vi "Set Gamma Adjust.vi"(8 "error in (no error)":errorcluster, 9 "Gamma Adjust":dbl=120.0, 10 "CAN Offset":u32=160 format="%x", 11 "interface object in":refnum<k20>) -> (0 "error out":errorcluster, 3 "interface object out":refnum<k20>)   [LabVIEW 2014]
uses:
  <vilib>/RioEmbeddedCAN/RioEmbeddedCAN.llb/CANWrite.vi
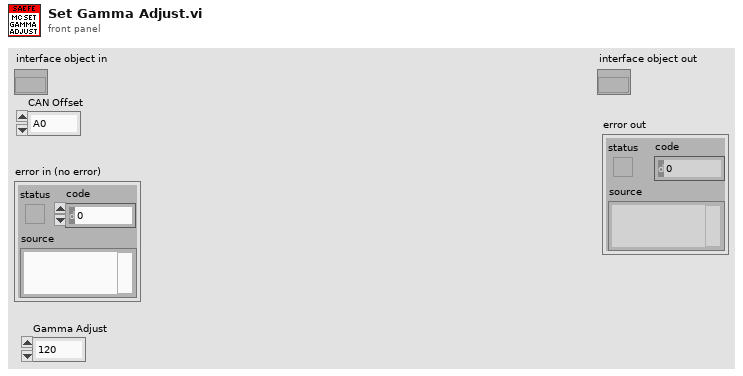
[diagram p1: front panel]
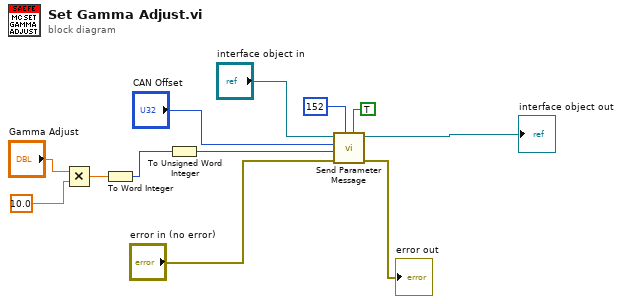
[diagram p0: block diagram]
diagram:
  n1 = Multiply(x="Gamma Adjust", y=10.0) -> (x*y=w4:dbl)
  n2 = To Word Integer(number=w4) -> (16bit integer=w2:i16)
  n3 = To Unsigned Word Integer(number=w2) -> (unsigned 16bit integer=w1:u16)
  n4 = call "Send Parameter Message.vi"("Write?"=TRUE, "Param Address"=i16 152, "error in (no error)"="error in (no error)", "Data"=w1, "CAN Offset"="CAN Offset", "interface object in"="interface object in") -> ("error out"=→"error out":errorcluster, "interface object out"=→"interface object out":refnum<k20>)  [unwired: 4 in]
